vi "Volume entry-Event handler-Proceed.vi"(11 "ROI Info":T1={"ROI Enum"=enum."Point", "Coordinates"=[], "Zoom"=0.0, "POI Dwell time"=1.0, "Rel. Resolution"=1.0, "Laser Power"=1.0, "Frame Size"=1.0, "FOV"=1.0, "Z start"=0.0, "Z stop"=0.0, "Z planeIdx(s)"=[], "Z planecodes(s)"=[]} {"FOV" min=1.0 max=10.0 step=1.0; "Frame Size" min=1.0 max=10.0 step=1.0; "Laser Power" min=1.0 max=10.0 step=0.10000000149011612; "Rel. Resolution" min=1.0 max=10.0 step=1.0; "POI Dwell time" min=1.0 max=10.0 step=0.10000000149011612; "Zoom" min=1.0 max=10.0 step=0.10000000149011612}) -> (2 "Zoom":dbl, 3 "ROI Info []":T1[](array[typedef]) {"FOV" min=1.0 max=10.0 step=1.0; "Frame Size" min=1.0 max=10.0 step=1.0; "Laser Power" min=1.0 max=10.0 step=0.10000000149011612; "Rel. Resolution" min=1.0 max=10.0 step=1.0; "POI Dwell time" min=1.0 max=10.0 step=0.10000000149011612; "Zoom" min=1.0 max=10.0 step=0.10000000149011612})   [LabVIEW 2020]
uses:
  Typedefs/ROI spec.ctl
  Typedefs/ROI ID Enum.ctl
  ROI Entry screen/Globals/gl_Volume Entry UI globals.vi
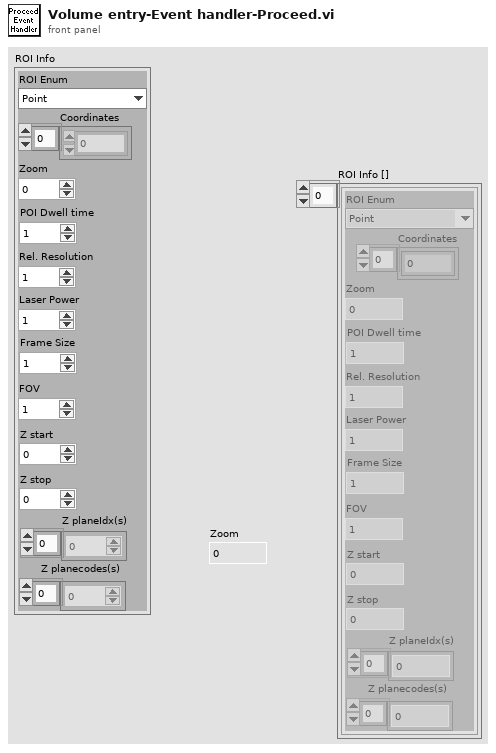
[diagram p1: front panel]
types:
  T1 = typedef "ROI spec.ctl" = cluster{"ROI Enum":T2, "Coordinates":i32[], "Zoom":dbl, "POI Dwell time":dbl, "Rel. Resolution":dbl, "Laser Power":dbl, "Frame Size":dbl, "FOV":dbl, "Z start":dbl, "Z stop":dbl, "Z planeIdx(s)":i32[], "Z planecodes(s)":u8[]}
  T2 = typedef "ROI ID Enum.ctl" = enum16{"Point", "MiniScan", "Comp. MiniScan", "Rectangle", "Comp. volume", "Arb. plane point", "None"}
  T3 = typedef "Volume entry ctrl refs cluster.ctl" = cluster{"Z-step (planes)":refnum<vi>, "Volume":refnum<vi>, "Dual Rectangle":refnum<vi>, "Zoom":refnum<vi>, "Z-plane 1":refnum<vi>, "Z-plane 2":refnum<vi>, "ZplaneIndex (zero based)":refnum<vi>}
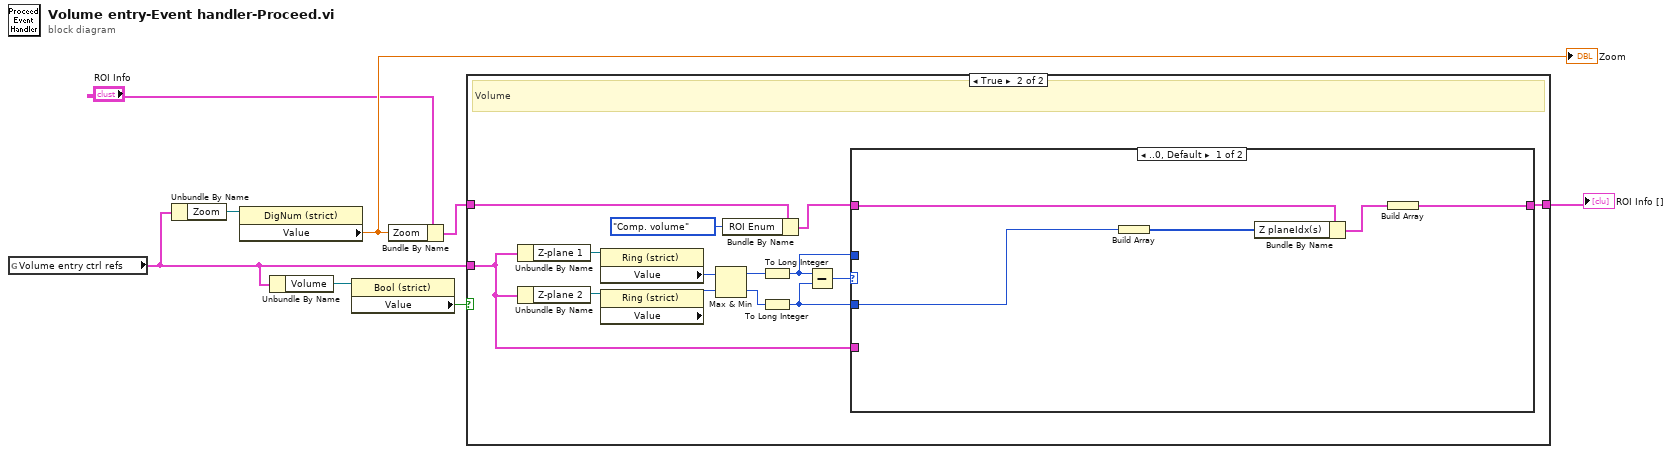
[diagram p0: block diagram]
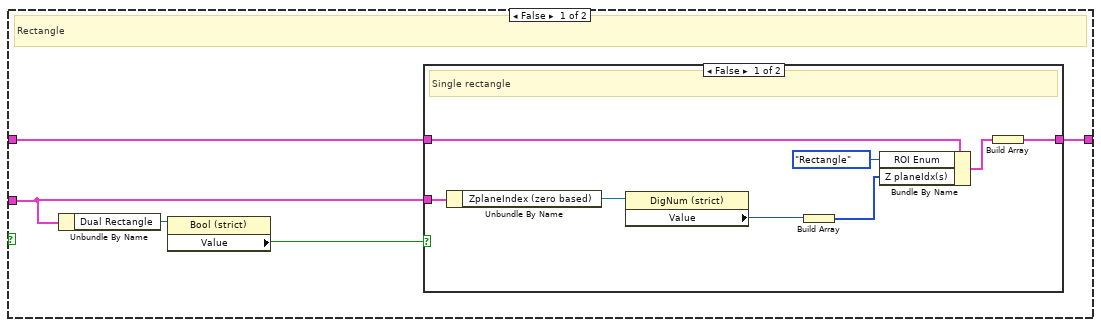
[diagram p2: hidden frame]
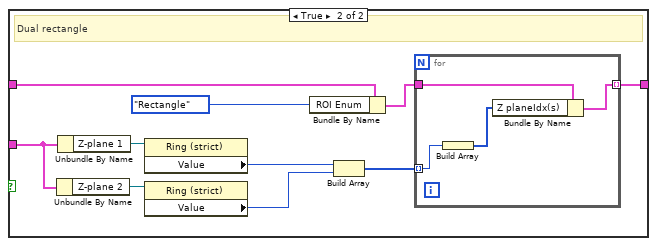
[diagram p3: hidden frame]
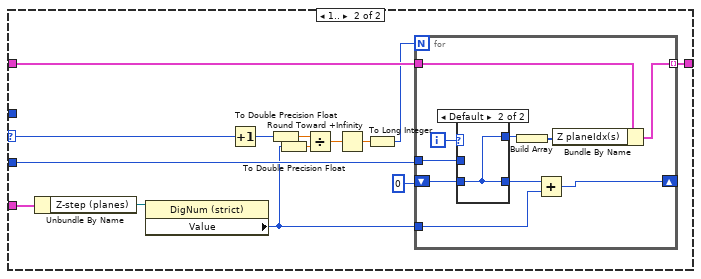
[diagram p4: hidden frame]
diagram:
  n1 = global read "gl_Volume Entry UI globals.vi" "Volume entry ctrl refs"() -> (w3:T3)
  n2 = Unbundle By Name(w3) -> ("Zoom"=w5:refnum<vi>)
  n3 = property on="Property Node" class="DigNum (strict)"(reference=w5) -> ("Value"=w6:dbl)  [unwired: 1 in, 2 out]
  "Zoom" <- w6
  n4 = Unbundle By Name(w3) -> ("Volume"=w7:refnum<vi>)
  n5 = property on="Property Node" class="Bool (strict)"(reference=w7) -> ("Value"=w8:bool)  [unwired: 1 in, 2 out]
  n6 = Bundle By Name(cluster="ROI Info", "Zoom"=w6) -> (w4:T1)
  n7 = case shown="True" w8 {
    tunnel: w4 -> [w12 w43]
    tunnel: [w13 w45] -> w1
    tunnel: w3 -> [w9 w36]
    frame False {
      # "Rectangle"
      n8 = Unbundle By Name(w9) -> ("Dual Rectangle"=w11:refnum<vi>)
      n9 = property class="Bool (strict)"(reference=w11) -> ("Value"=w10:bool)  [unwired: 1 in, 2 out]
      n10 = case shown="False" w10 {
        tunnel: [w21 w27] -> w13
        tunnel: w12 -> [w20 w28]
        tunnel: w9 -> [w16 w26]
        frame False {
          # "Single rectangle"
          n11 = Unbundle By Name(w16) -> ("ZplaneIndex (zero based)"=w17:refnum<vi>)
          n12 = property on="Property Node" class="DigNum (strict)"(reference=w17) -> ("Value"=w15:i32)  [unwired: 1 in, 2 out]
          n13 = Build Array(w15) -> (w14:i32[])
          n14 = Bundle By Name(cluster=w20, "ROI Enum"=ROI_ID_Enum."Rectangle", "Z planeIdx(s)"=w14) -> (w19:T1)
          n15 = Build Array(w19) -> (w21:T1[])
        }
        frame True {
          # "Dual rectangle"
          n16 = Unbundle By Name(w26) -> ("Z-plane 2"=w23:refnum<vi>)
          n17 = Unbundle By Name(w26) -> ("Z-plane 1"=w22:refnum<vi>)
          n18 = property class="Ring (strict)"(reference=w22) -> ("Value"=w25:u16)  [unwired: 1 in, 2 out]
          n19 = property class="Ring (strict)"(reference=w23) -> ("Value"=w24:u16)  [unwired: 1 in, 2 out]
          n20 = Bundle By Name(cluster=w28, "ROI Enum"=ROI_ID_Enum."Rectangle") -> (w30:T1)
          n21 = Build Array(w25, w24) -> (w31:u16[])
          n22 = for {
            tunnel: w30 -> [w35]
            tunnel: w31 -> [w33] mode=indexing
            tunnel: [w34] -> w27 mode=indexing
            n23 = Build Array(w33) -> (w32:u16[])
            n24 = Bundle By Name(cluster=w35, "Z planeIdx(s)"=w32) -> (w34:T1)
          }
        }
      }
    }
    frame True {
      # "Volume"
      n25 = Unbundle By Name(w36) -> ("Z-plane 1"=w40:refnum<vi>)
      n26 = Unbundle By Name(w36) -> ("Z-plane 2"=w39:refnum<vi>)
      n27 = property class="Ring (strict)"(reference=w40) -> ("Value"=w38:u16)  [unwired: 1 in, 2 out]
      n28 = property class="Ring (strict)"(reference=w39) -> ("Value"=w37:u16)  [unwired: 1 in, 2 out]
      n29 = Max & Min(x=w38, y=w37) -> (max(x,y)=w49:u16, min(x,y)=w48:u16)
      n30 = Bundle By Name(cluster=w43, "ROI Enum"=ROI_ID_Enum."Comp. volume") -> (w42:T1)
      n31 = To Long Integer(number=w49) -> (32bit integer=w47:i32)
      n32 = To Long Integer(number=w48) -> (32bit integer=w46:i32)
      n33 = Subtract(x=w47, y=w46) -> (x-y=w41:i32)
      n34 = case shown="..0, Default" w41 {
        selector: w41 -> [_ w68]
        tunnel: w47 -> [_ _]
        tunnel: w46 -> [w50 w67]
        tunnel: w42 -> [w53 w65]
        tunnel: [w54 w64] -> w45
        tunnel: w36 -> [_ w57]
        frame ..0, Default {
          n35 = Build Array(w50) -> (w51:i32[])
          n36 = Bundle By Name(cluster=w53, "Z planeIdx(s)"=w51) -> (w52:T1)
          n37 = Build Array(w52) -> (w54:T1[])
        }
        frame 1.. {
          n38 = Unbundle By Name(w57) -> ("Z-step (planes)"=w59:refnum<vi>)
          n39 = property class="DigNum (strict)"(reference=w59) -> ("Value"=w58:i32)  [unwired: 1 in, 2 out]
          n40 = Increment(x=w68) -> (x+1=w63:i32)
          n41 = To Double Precision Float(number=w63) -> (double precision float=w56:dbl)
          n42 = To Double Precision Float(number=w58) -> (double precision float=w55:dbl)
          n43 = Divide(x=w56, y=w55) -> (x/y=w62:dbl)
          n44 = Round Toward +Infinity(x=w62) -> (ceil(x): smallest int >= x=w61:dbl)
          n45 = To Long Integer(number=w61) -> (32bit integer=w60:i32)
          n46 = for {
            N: w60 -> [_]
            tunnel: w67 -> [w77]
            shift-right: [w72] -> _
            shift-left: 0 -> [w76]
            tunnel: w65 -> [w75]
            tunnel: [w74] -> w64 mode=indexing
            tunnel: w58 -> [w71]
            i -> [w78]
            n47 = case shown="Default" w78 {
              tunnel: w77 -> [w79 _]
              tunnel: [w79 w80] -> w70
              tunnel: [w79 w80] -> w73
              tunnel: w76 -> [_ w80]
              frame 0 {
              }
              frame Default {
              }
            }
            n48 = Build Array(w70) -> (w69:i32[])
            n49 = Add(x=w73, y=w71) -> (x+y=w72:i32)
            n50 = Bundle By Name(cluster=w75, "Z planeIdx(s)"=w69) -> (w74:T1)
          }
        }
      }
    }
  }
  "ROI Info []" <- w1
